vi "SampleDataInfo.vi"(9 "clSampleData":T2 {"Timestamp" format="%.6f"}, 10 "clConfig":T1={"F0"=60, "SettlingTime"=7.0, "AnalysisCycles"=20.0, "SampleRate"=4800.0, "NumChannels"=6, "TsOffset"=enum."start"}) -> (1 "LastTS":ext format="%.6f", 2 "FirstTS":ext format="%.6f", 4 "iActualPts":u32)   [LabVIEW 2014, in "AnalysisPlugins.lvlib" / "AnalysisPluginsBase.lvclass"]
uses:
  AnalysisPluginsBase.lvclass
  Typedefs/clSampleData.ctl
  Typedefs/clAnalysisConfig.ctl
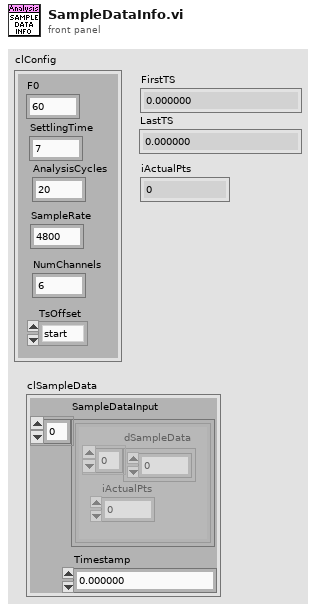
[diagram p1: front panel]
types:
  T1 = typedef "AnalysisPlugins.lvlib/AnalysisPluginsBase.lvclass/clAnalysisConfig.ctl" = cluster{"F0":u32, "SettlingTime":dbl, "AnalysisCycles":dbl, "SampleRate":dbl, "NumChannels":u32, "TsOffset":enum16{"start", "middle", "end"}}
  T2 = typedef "AnalysisPlugins.lvlib/AnalysisPluginsBase.lvclass/clSampleData.ctl" = cluster{"Timestamp":ext, "SampleDataInput":cluster{"dSampleData":dbl[], "iActualPts":i32}[]}
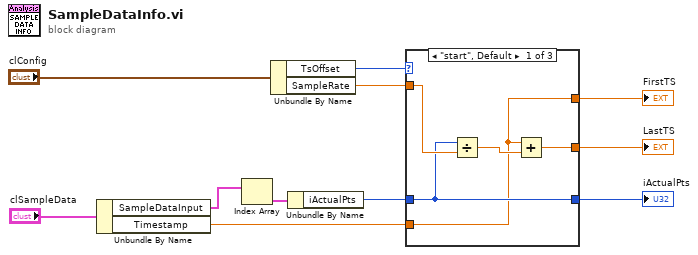
[diagram p0: block diagram]
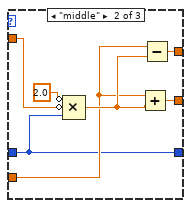
[diagram p2: hidden frame]
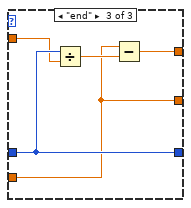
[diagram p3: hidden frame]
diagram:
  n1 = Unbundle By Name("clSampleData") -> ("SampleDataInput"=w9:cluster{"dSampleData":dbl[], "iActualPts":i32}[], "Timestamp"=w7:ext)
  n2 = Index Array(array=w9) -> (element=w8:cluster{"dSampleData":dbl[], "iActualPts":i32})  [unwired: 1 in]
  n3 = Unbundle By Name("clConfig") -> ("TsOffset"=w6:enum16{"start", "middle", "end"}, "SampleRate"=w4:dbl)
  n4 = Unbundle By Name(w8) -> ("iActualPts"=w5:i32)
  n5 = case shown="\"start\", Default" w6 {
    tunnel: w7 -> [w12 w18 w24]
    tunnel: w5 -> [w15 w17 w28]
    tunnel: w4 -> [w16 w23 w27]
    tunnel: [w12 w21 w26] -> w3
    tunnel: [w13 w20 w24] -> w2
    tunnel: [w15 w17 w28] -> w1
    frame "start", Default {
      n6 = Divide(x=w15, y=w16) -> (x/y=w14:dbl)
      n7 = Add(x=w12, y=w14) -> (x+y=w13:ext)
    }
    frame "middle" {
      n8 = Compound Arithmetic op=MULTIPLY(invert 2.0 ("value"), invert w23, w17) -> (w19:dbl)
      n9 = Add(x=w18, y=w19) -> (x+y=w20:ext)
      n10 = Subtract(x=w18, y=w19) -> (x-y=w21:ext)
    }
    frame "end" {
      n11 = Divide(x=w28, y=w27) -> (x/y=w25:dbl)
      n12 = Subtract(x=w24, y=w25) -> (x-y=w26:ext)
    }
  }
  "FirstTS" <- w3
  "LastTS" <- w2
  "iActualPts" <- w1
